vi "Telnet Read.vi"(4 "line separator":string, 5 "read mode (normal)":enum16{"normal", "line", "buffered"}(ring), 6 "error in (no error)":errorcluster, 7 "timeout ms (25000)":i32=25000, 8 "bytes to read":i32=60, 9 "telnet connection":T2) -> (0 "error out":errorcluster, 2 "data out":string, 3 "telnet connection out":T2)   [LabVIEW 2015]
doc: "Reads data from a connection opened with Telent Open Connection and filters out all Telnet Escape Sequences.\n\nread mode:\n normal (same as TCP Read)\n line (returns data up to (and including) the line separator)\n buffered (only returns data if the requeste number of bytes is available)"
uses:
  Telnet Session.ctl
  Semaphore RefNum.ctl
panel:
  out "Length":i32
  in  "semaphore":T1
  in  "Safety Mode On (FALSE)":bool=TRUE
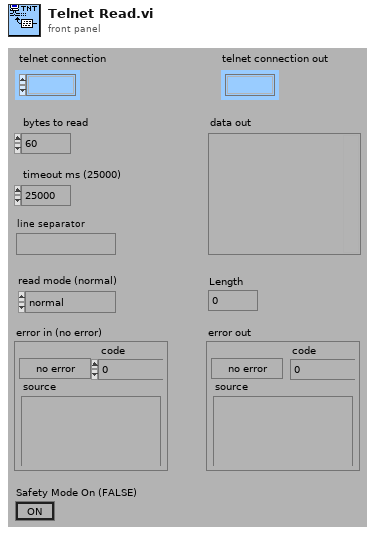
[diagram p1: front panel]
types:
  T1 = typedef "Semaphore RefNum.ctl" = refnum<k1>
  T2 = typedef "Telnet Session.ctl" = refnum<k1>
  T3 = enum16{"reset", "register", "get data", "set data", "unregister", "test", "get objects"}
  T4 = cluster{"bytes to read":i32, "timeout ms (25000)":i32, "read mode (normal)":enum16{"normal", "line", "buffered"}, "line separator":string}
  T5 = typedef "Telnet Connection Data.ctl" = cluster{"id":refnum<k5>, "read sem":T1, "write sem":T1, "read buffer":string, "read unfiltered buffer":string}
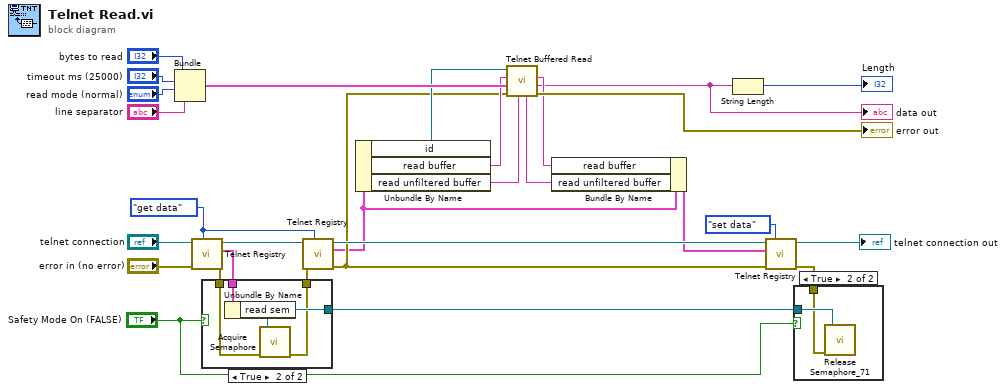
[diagram p0: block diagram]
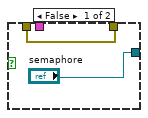
[diagram p3: hidden frame]
diagram:
  w9 = T3."get data" ("function (get data)")
  n1 = Bundle("bytes to read"="bytes to read", "timeout ms (25000)"="timeout ms (25000)", "read mode (normal)"="read mode (normal)", "line separator"="line separator") -> (w27:T4)  [unwired: 1 in]
  n2 = call "Telnet Registry.vi"("function (get data)"=w9, "error in (no error)"="error in (no error)", "object"="telnet connection") -> ("error out"=w17:errorcluster, "object data"=w15:T5, "object out"=w16:T2)  [unwired: 4 in, 2 out]
  n3 = case shown="True" "Safety Mode On (FALSE)" {
    tunnel: ["semaphore" w35] -> w18
    tunnel: w17 -> [w31 w34]
    tunnel: w15 -> [_ w33]
    tunnel: [w31 w32] -> w13
    frame False {
    }
    frame True {
      n4 = Unbundle By Name(w33) -> ("read sem"=w35:T1)
      n5 = call <vilib>:"Acquire Semaphore.vi"("error in (no error)"=w34, "semaphore"=w35) -> ("error out"=w32:errorcluster)  [unwired: 3 in, 2 out]
    }
  }
  n6 = call "Telnet Registry.vi"("function (get data)"=w9, "error in (no error)"=w13, "object"=w16) -> ("error out"=w8:errorcluster, "object data"=w4:T5, "object out"=w14:T2)  [unwired: 4 in, 2 out]
  n7 = Unbundle By Name(w4) -> ("id"=w25:refnum<k5>, "read buffer"=w24:string, "read unfiltered buffer"=w22:string)
  n8 = call "Telnet Buffered Read.vi"("unfiltered buffer in"=w22, "error in (no error)"=w8, "read info"=w27, "buffer in"=w24, "connection ID"=w25) -> ("error out"=→"error out":errorcluster, "data"=w2:string, "buffer out"=w23:string, "unfiltered buffer out"=w21:string)  [unwired: 2 in, 1 out]
  "data out" <- w2
  n9 = Bundle By Name(cluster=w4, "read buffer"=w23, "read unfiltered buffer"=w21) -> (w3:T5)
  n10 = String Length(string=w2) -> (length=→"Length":i32)
  n11 = call "Telnet Registry.vi"("function (get data)"=T3."set data", "error in (no error)"=w8, "object data in"=w3, "object"=w14) -> ("error out"=w12:errorcluster, "object out"=→"telnet connection out":T2)  [unwired: 3 in, 3 out]
  n12 = case shown="True" "Safety Mode On (FALSE)" {
    tunnel: w18 -> [_ w37]
    tunnel: w12 -> [_ w36]
    frame False {
    }
    frame True {
      n13 = call <vilib>:"Release Semaphore_71.vi"("error in (no error)"=w36, "semaphore"=w37) -> ()  [unwired: 4 in, 2 out]
    }
  }
